vi "stop receiver loop.vi"(8 "error in":errorcluster, 11 "receiver reference":T1) -> (0 "error out":errorcluster)   [LabVIEW 2013, in "lvnano.lvlib"]
uses:
  lvnano.lvlib
  receive loop reference.ctl
  lvnanomsg.dll
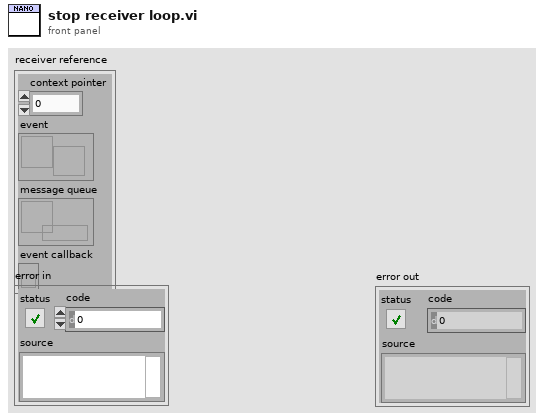
[diagram p1: front panel]
types:
  T1 = typedef "lvnano.lvlib/receive loop reference.ctl" = cluster{"context pointer":i64, "event":refnum<user-event>, "message queue":refnum<queue>, "event callback":refnum<k27>}
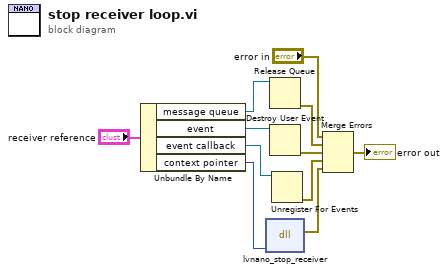
[diagram p0: block diagram]
diagram:
  n1 = Unbundle By Name("receiver reference") -> ("message queue"=w8:refnum<queue>, "event"=w9:refnum<user-event>, "event callback"=w10:refnum<k27>, "context pointer"=w1:i64)
  n2 = dll-call lib="C:/Users/Daniel/Documents/nanomsg/lvnano/lvnanomsg.dll" fn="lvnano_stop_receiver"("rthread context"=w1) -> (error out=w6:errorcluster)  [unwired: 5 in, 1 out]
  n3 = Release Queue(queue=w8) -> (error out=w3:errorcluster)  [unwired: 2 in, 2 out]
  n4 = Destroy User Event(user event=w9) -> (error out=w2:errorcluster)  [unwired: 1 in]
  n5 = Unregister For Events(event registration refnum=w10) -> (error out=w7:errorcluster)  [unwired: 1 in]
  n6 = Merge Errors("error in", w3, w2, w7, w6) -> (→"error out":errorcluster)
